vi "AxisReadValues.vi"(1 "AxisNo":u16) -> (0 "AxisReadValuesOUT":T1)   [LabVIEW 2020, in "SMCD14_lib.lvlib"]
uses:
  AxisReadValues_typedef.ctl
  Globals.vi
  SMCD14_lib.lvlib
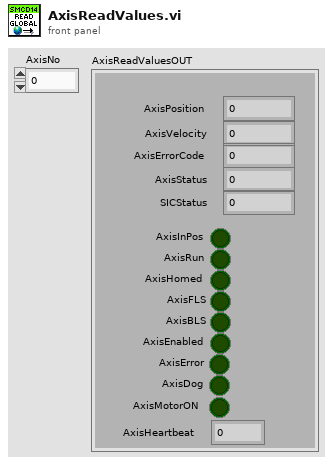
[diagram p1: front panel]
types:
  T1 = typedef "SMCD14_lib.lvlib/AxisReadValues_typedef.ctl" = cluster{"AxisPosition":dbl, "AxisStatus":i16, "AxisErrorCode":i16, "AxisInPos":bool, "AxisRun":bool, "AxisHomed":bool, "AxisFLS":bool, "AxisBLS":bool, "AxisEnabled":bool, "AxisError":bool, "AxisDog":bool, "AxisVelocity":dbl, "AxisHeartbeat":i16, "SICStatus":i16, "AxisMotorON":bool}
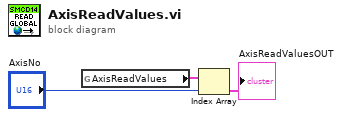
[diagram p0: block diagram]
diagram:
  n1 = global read "Globals.vi" "AxisReadValues"() -> (w2:T1[])
  n2 = Index Array(array=w2, index="AxisNo") -> (element=→"AxisReadValuesOUT":T1)
